vi "Has Refresh Token.vi"(11 "Async Authorization in":refnum<class "Async Authorization.lvclass">) -> (2 "Has Refresh Token":bool)   [LabVIEW 2020, in "OAuth2.lvlib" / "Async Authorization.lvclass"]
uses:
  Async Authorization.lvclass
  Authorization/Authorization.lvclass
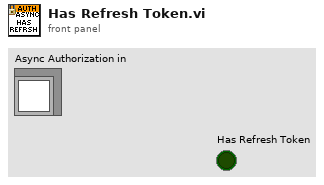
[diagram p1: front panel]
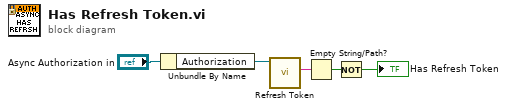
[diagram p0: block diagram]
diagram:
  n1 = Unbundle By Name("Async Authorization in") -> ("Authorization"=w4:refnum<class "Authorization.lvclass">)
  n2 = call "Refresh Token.vi"("Authorization in"=w4) -> ("Refresh Token"=w3:string)  [unwired: 10 in]
  n3 = Empty String/Path?(string/path=w3) -> (empty?=w2:bool)
  n4 = Not(x=w2) -> (.not. x?=→"Has Refresh Token":bool)
